vi "APS wait field bus error int motion.vi"(8 "error in (no error)":errorcluster caption="错误输入（无错误）", 10 "Time_Out":i32, 11 "Axis_ID":i32) -> (0 "error out":errorcluster caption="错误输出", 3 "function return":i32)   [LabVIEW 2011, in "APS168.lvlib"]
doc: "I32 FNTYPE APS_wait_field_bus_error_int_motion( I32 Axis_ID, I32 Time_Out );"
uses:
  APS168.lvlib
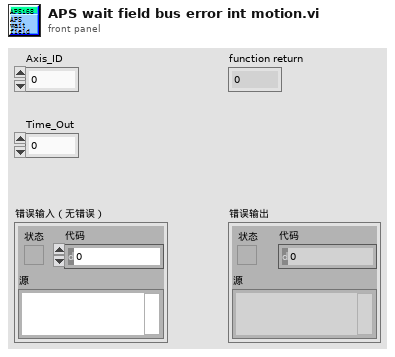
[diagram p1: front panel]
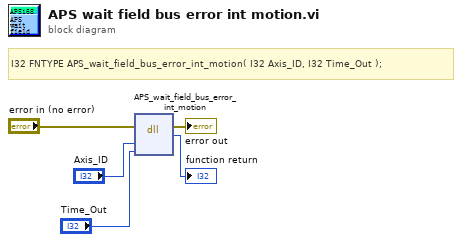
[diagram p0: block diagram]
diagram:
  # "I32 FNTYPE APS_wait_field_bus_error_int_motion( I32 Axis_ID, I32 Time_Out );"
  n1 = dll-call lib="PTH1Labs E软件ADLINK 204CAPS_1_7_1_LIB line 连续运动204APS168.*" fn="APS_wait_field_bus_error_int_motion"(error in="error in (no error)", "Axis_ID"="Axis_ID", "Time_Out"="Time_Out") -> (error out=→"error out":errorcluster, →"function return":i32)  [unwired: 4 in, 1 out]
